vi "Read datatype.vi"(8 "error in (no error)":errorcluster, 11 "JSON Numeric in":refnum<class "JSON Numeric.lvclass">) -> (0 "error out":errorcluster, 2 "datatype":T1, 3 "JSON Numeric out":refnum<class "JSON Numeric.lvclass">)   [LabVIEW 2015, in "LVJSON.lvlib" / "JSON Numeric.lvclass"]
uses:
  JSON Numeric.lvclass
  JSON Types.ctl
  LVJSON.lvlib
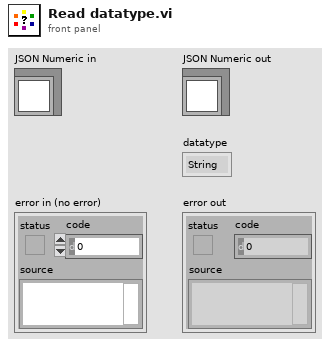
[diagram p1: front panel]
types:
  T1 = typedef "LVJSON.lvlib/JSON Types.ctl" = enum16{"String", "Numeric", "Boolean", "NULL", "Object", "1D Array", "Unknown"}
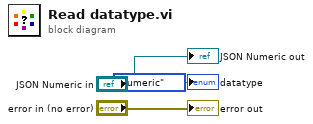
[diagram p0: block diagram]
diagram:
  "error out" <- "error in (no error)"
  "JSON Numeric out" <- "JSON Numeric in"
  "datatype" <- JSON_Types."Numeric" ("datatype")
